vi "Write Passed.vi"(8 "error in (no error)":errorcluster, 10 "Passed?":bool, 11 "Assertion Result In":refnum<class "Assertion Result.lvclass">) -> (0 "error out":errorcluster, 3 "Assertion Result Out":refnum<class "Assertion Result.lvclass">)   [LabVIEW 2020, in "Assertion Result.lvclass"]
uses:
  Assertion Result.lvclass
  Public/TypeDefs/Status.ctl
  Assertion Result.lvclass/Assertion Result.ctl
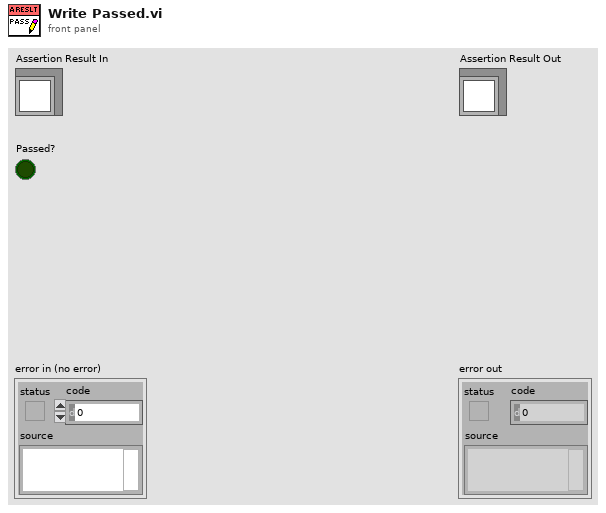
[diagram p1: front panel]
types:
  T1 = typedef "Assertion Result.lvclass/Status.ctl" = enum16{"Pass", "Fail", "Error", "Skipped", "Setup Error", "Broken", "Teardown Error"}
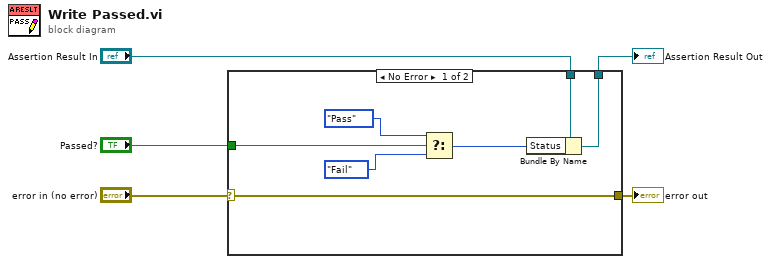
[diagram p0: block diagram]
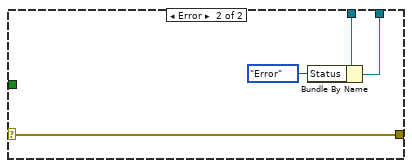
[diagram p2: hidden frame]
diagram:
  n1 = case shown="No Error" "error in (no error)" {
    selector: "error in (no error)" -> [w6 w13]
    tunnel: "Assertion Result In" -> [w12 w16]
    tunnel: [w11 w15] -> w4
    tunnel: "Passed?" -> [w10 _]
    tunnel: [w6 w13] -> w1
    frame No Error {
      n2 = Select(t=Status."Pass" ("Status"), s=w10, f=Status."Fail") -> (s? t:f=w9:T1)
      n3 = Bundle By Name(cluster=w12, "Status"=w9) -> (w11:refnum<class "Assertion Result.lvclass">)
    }
    frame Error {
      n4 = Bundle By Name(cluster=w16, "Status"=Status."Error") -> (w15:refnum<class "Assertion Result.lvclass">)
    }
  }
  "error out" <- w1
  "Assertion Result Out" <- w4
